vi "Variable.vi"(7 "VariableName":string, 8 "InformIgor":bool, 9 "Sequence":bool, 10 "SequenceFunction":string, 11 "DefaultValue":dbl format="%^#_6g") -> (3 "Variable":refnum<class "Variable.lvclass">)   [LabVIEW 2013, in "VariableManagerAPI.lvlib"]
doc: "Return Variable definition object.\nThe object contains given values (optional).\nData can be accessed through property node.\n\n<B>VariableName</B>: the name of the variable\n<B>DefaultValue</B>: the evaluated value of the variable when sequence is false.\n<B>SequenceFunction</B>: the evaluated value of the variable when sequence is true.\n<B>Sequence</B>: the boolean determine how the variable is evaluated.\n<B>InformIgor</B>: the boolean determine if the variable value must be informed to Igor."
uses:
  VariableManagerAPI.lvlib
  Variable/Variable.lvclass
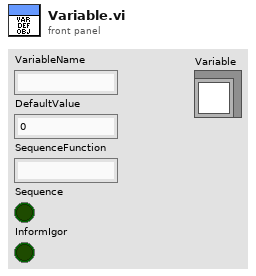
[diagram p1: front panel]
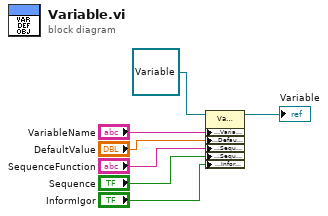
[diagram p0: block diagram]
diagram:
  n1 = property class="Variable.lvclass"(reference=refnum<class "Variable.lvclass"> refnum ("Variable.lvclass"), "Accessors:VariableName"="VariableName", "Accessors:DefaultValue"="DefaultValue", "Accessors:SequenceFunction"="SequenceFunction", "Accessors:Sequence"="Sequence", "Accessors:InformIgor"="InformIgor") -> (reference out=→"Variable":refnum<class "Variable.lvclass">)  [unwired: 1 in, 1 out]
